vi "get Session Name.vi"(0 "OBJ - Session in":refnum<class "Session - Root.lvclass">, 11 "error in (no error)":errorcluster) -> (4 "OBJ - Session out":refnum<class "Session - Root.lvclass">, 6 "Session Name":string, 15 "error out":errorcluster)   [LabVIEW 2015, in "Session - Root.lvclass"]
doc: "Extracts named notifier; typically to release or destroy reference"
uses:
  Session - Root.lvclass
  Session - Root.lvclass/Session - Root.ctl
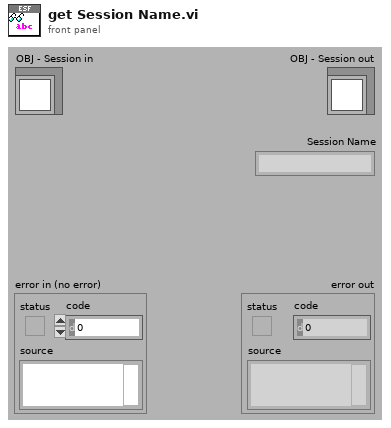
[diagram p1: front panel]
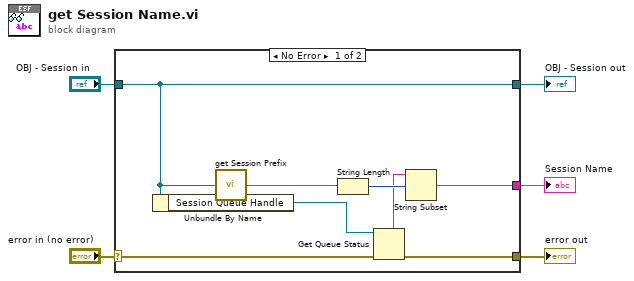
[diagram p0: block diagram]
diagram:
  n1 = case shown="No Error" "error in (no error)" {
    selector: "error in (no error)" -> [w13 w14]
    tunnel: [w12 w14] -> w4
    tunnel: [w7 w15] -> w2
    tunnel: "OBJ - Session in" -> [w7 w15]
    tunnel: [w8 _] -> w1
    frame No Error {
      n2 = Unbundle By Name(w7) -> ("Session Queue Handle"=w11:refnum<queue>)
      n3 = call-dynamic "get Session Prefix.vi"("Session - Root"=w7) -> ("Session Prefix"=w6:string)  [unwired: 14 in]
      n4 = String Length(string=w6) -> (length=w10:i32)
      n5 = Get Queue Status(queue=w11, error in (no error)=w13) -> (queue name=w9:string, error out=w12:errorcluster)  [unwired: 1 in, 6 out]
      n6 = String Subset(string=w9, offset (0)=w10) -> (substring=w8:string)  [unwired: 1 in]
    }
    frame Error {
    }
  }
  "error out" <- w4
  "OBJ - Session out" <- w2
  "Session Name" <- w1
